vi "AuxStabilizeMW.vi"(0 "PowerStableSettings":refnum<vi>, 3 "error in":errorcluster) -> (10 "error out":errorcluster)   [LabVIEW 2017]
uses:
  controls/PowerStableSettings.ctl
  controls/AgilentCtrlEnum.ctl
  <vilib>/Analysis/baseanly.llb/Mean (DBL).vi
  <vilib>/Analysis/NI_AALBase.lvlib
panel:
  out "coerced(x)":dbl
  out "upper limit":dbl
  in  "target power":dbl format="%#_13g"
  out "Array":dbl[](array[numeric])
  out "mean":dbl format="%0.4f"
  in  "RSNRPZ visa":refnum<visa-resource-name> caption="VISA resource name"
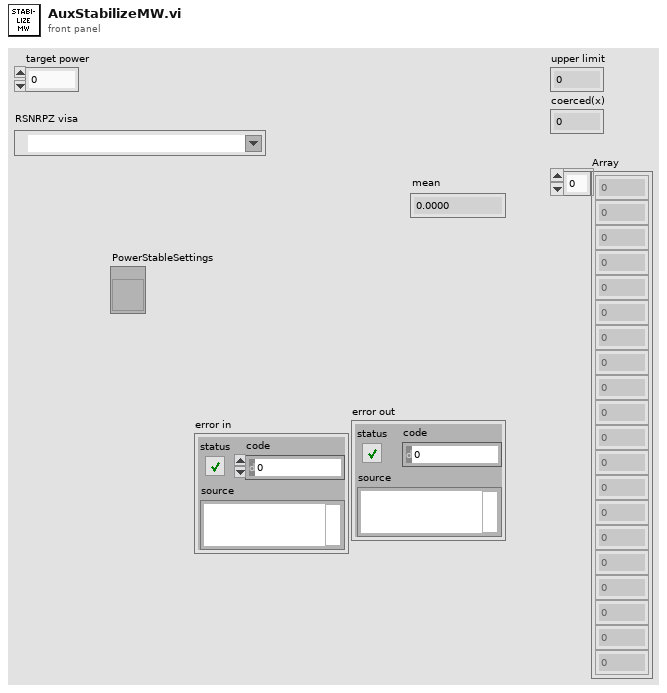
[diagram p1: front panel]
types:
  T1 = typedef "AgilentCtrlEnum.ctl" = enum16{"WRITE_POW", "READ_POW"}
  T2 = typedef "PowerStableSettings.ctl" = cluster{"Lock Power":bool, "Number measurements":i32, "Min AWG Power [dBm] :":dbl, "Max AWG Power [dBm] :":dbl, "Min Power Difference [dBm] : ":dbl, "Max Power Difference [dBm] :":dbl, "Agilient visa ":string}
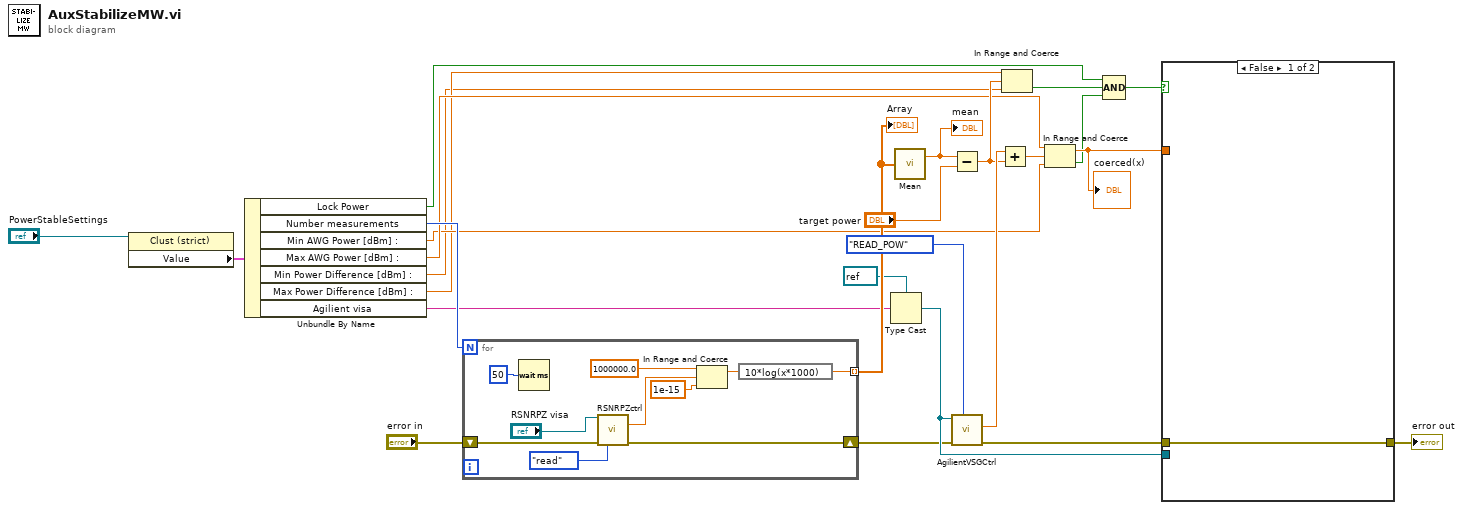
[diagram p0: block diagram]
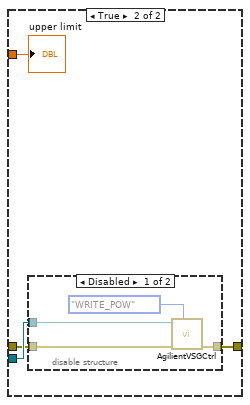
[diagram p2: hidden frame]
diagram:
  n1 = property class="Clust (strict)"(reference="PowerStableSettings") -> ("Value"=w14:T2)  [unwired: 1 in, 2 out]
  n2 = Unbundle By Name(w14) -> ("Lock Power"=w13:bool, "Number measurements"=w12:i32, "Min AWG Power [dBm] :"=w10:dbl, "Max AWG Power [dBm] :"=w11:dbl, "Min Power Difference [dBm] :"=w8:dbl, "Max Power Difference [dBm] :"=w9:dbl, "Agilient visa"=w6:string)
  n3 = for {
    N: w12 -> [_]
    tunnel: [w29] -> w26 mode=indexing
    shift-right: [w27] -> w3
    shift-left: "error in" -> [w28]
    n4 = Wait (ms)(milliseconds to wait=u32 50) -> ()  [unwired: 1 out]
    n5 = call "RSNRPZctrl.vi"("VISA session in"="RSNRPZ visa", "error in (no error)"=w28, "action"=enum16{"close", "update", "read", "init"}."read") -> ("Measurement"=w33:dbl, "error out"=w27:errorcluster)  [unwired: 9 in, 2 out]
    n6 = In Range and Coerce(upper limit=1000000.0, x=w33, lower limit=1e-15) -> (coerced(x)=w30:dbl)  [unwired: 1 out]
    n7 = expression code="10*log(x*1000)"(w30) -> (w29:dbl)
  }
  "Array" <- w26
  n8 = Type Cast(type=refnum<visa-resource-name> refnum ("VISA resource name"), x=w6) -> (*(type *) &x=w5:refnum<visa-resource-name>)
  n9 = call-poly <vilib>:"Mean.vi"("X"=w26) -> ("mean"=w16:dbl)  [unwired: 1 out]
  "mean" <- w16
  n10 = Subtract(x=w16, y="target power") -> (x-y=w23:dbl)
  n11 = call "AgilientVSGCtrl.vi"("action"=AgilentCtrlEnum."READ_POW", "error in (no error)"=w3, "VISA resource name"=w5) -> ("error out"=w2:errorcluster, "pow read"=w24:dbl)  [unwired: 7 in]
  n12 = Add(x=w24, y=w23) -> (x+y=w22:dbl)
  n13 = In Range and Coerce(upper limit=w9, x=w23, lower limit=w8) -> (In Range?=w19:bool)  [unwired: 1 out]
  n14 = In Range and Coerce(upper limit=w11, x=w22, lower limit=w10) -> (coerced(x)=w21:dbl, In Range?=w20:bool)
  "coerced(x)" <- w21
  n15 = Compound Arithmetic op=AND(w13, w19, w20) -> (w18:bool)
  n16 = case shown="False" w18 {
    tunnel: w21 -> [_ w40]
    tunnel: w5 -> [_ w41]
    tunnel: w2 -> [w37 w39]
    tunnel: [w37 w38] -> w1
    frame False {
    }
    frame True {
      n17 = disable-structure shown="Disabled" {
        disable-tunnel: w41 -> [w45 _]
        disable-tunnel: w39 -> [w43 _]
        disable-tunnel: [w42 _] -> w38
        frame Disabled {
          n18 = call "AgilientVSGCtrl.vi"("action"=AgilentCtrlEnum."WRITE_POW", "error in (no error)"=w43, "VISA resource name"=w45) -> ("error out"=w42:errorcluster)  [unwired: 7 in, 1 out]
        }
        frame Enabled {
        }
      }
      "upper limit" <- w40
    }
  }
  "error out" <- w1
